vi "CoMP-S Logging To Text File.vi"(8 "error in (no error)":errorcluster, 9 "Oversizing":bool, 11 "Input text":string) -> (0 "error out":errorcluster)   [LabVIEW 2014]
panel:
  out "size (in bytes)":i64
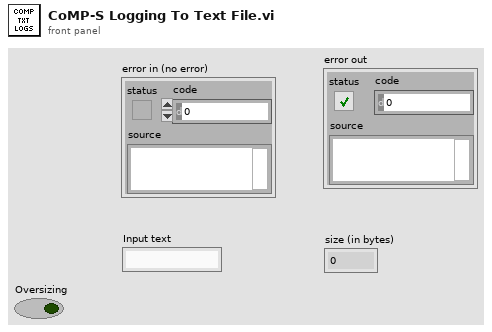
[diagram p1: front panel]
types:
  T1 = enum16{"open", "replace", "create", "open or create", "replace or create", "replace or create with confirmation"}
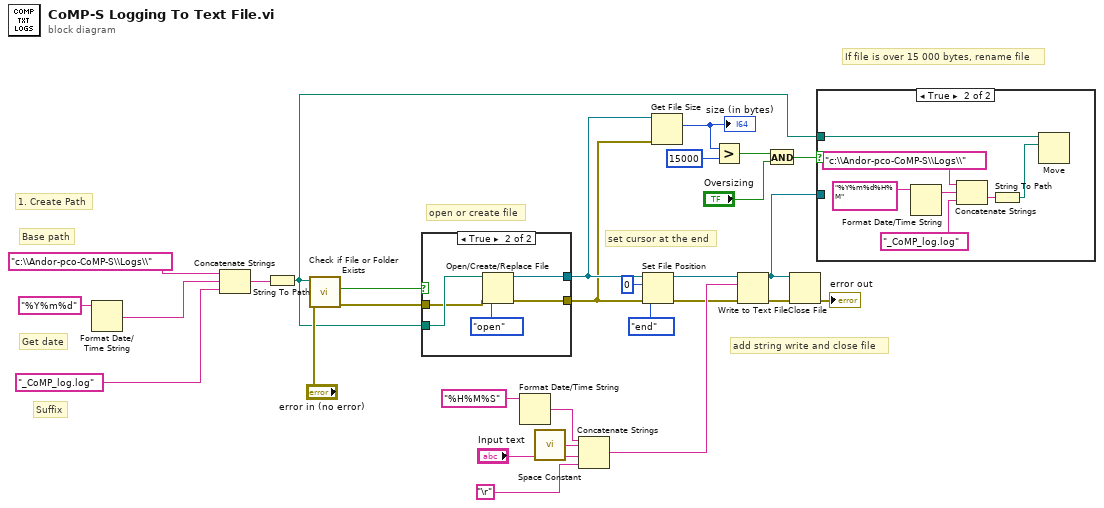
[diagram p0: block diagram]
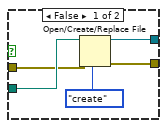
[diagram p3: hidden frame]
diagram:
  # "If file is over 15 000 bytes, rename file"
  # "set cursor at the end"
  # "open or create file"
  # "Suffix"
  # "1. Create Path"
  # "Get date"
  # "Base path"
  # "add string write and close file"
  n1 = Format Date/Time String(time format string (%c)="%Y%m%d") -> (date/time string=w4:string)  [unwired: 2 in]
  n2 = Concatenate Strings("c:\\Andor-pco-CoMP-S\\Logs\\" ("time format string (%c)"), w4, "_CoMP_log.log") -> (w26:string)
  n3 = String To Path(string=w26) -> (path=w9:path)
  n4 = call <vilib>:"Check if File or Folder Exists.vi"("error in (no error)"="error in (no error)", "path"=w9) -> ("error out"=w17:errorcluster, "file or folder exists?"=w25:bool)  [unwired: 7 in, 1 out]
  n5 = case shown="True" w25 {
    tunnel: w9 -> [w34 w38]
    tunnel: [w33 w37] -> w14
    tunnel: [w31 w36] -> w13
    tunnel: w17 -> [w30 w35]
    frame False {
      n6 = Open/Create/Replace File(file path (use dialog)=w34, error in=w30, operation (0:open)=T1."create") -> (refnum out=w33:refnum<file>, error out=w31:errorcluster)  [unwired: 3 in, 1 out]
    }
    frame True {
      n7 = Open/Create/Replace File(file path (use dialog)=w38, error in=w35, operation (0:open)=T1."open") -> (refnum out=w37:refnum<file>, error out=w36:errorcluster)  [unwired: 3 in, 1 out]
    }
  }
  n8 = Format Date/Time String(time format string (%c)="%H%M%S") -> (date/time string=w2:string)  [unwired: 2 in]
  n9 = call <vilib>:"Space Constant.vi"() -> ("String"=w1:string)
  n10 = Concatenate Strings(w2, w1, "Input text", "\r") -> (w19:string)
  n11 = Set File Position(offset (in bytes) (0)=i64 0, refnum=w14, from (0:start)=enum16{"start", "end", "current"}."end", error in=w13) -> (refnum out=w24:refnum<file>, error out=w18:errorcluster)
  n12 = Get File Size(file=w14, error in=w13) -> (size (in bytes)=w12:i64)  [unwired: 2 out]
  "size (in bytes)" <- w12
  n13 = Greater?(x=w12, y=i64 15000) -> (0:w8:bool)
  n14 = Write to Text File(file (use dialog)=w24, text=w19, error in=w18) -> (refnum out=w10:refnum<file>, error out=w29:errorcluster)  [unwired: 1 in, 1 out]
  n15 = And(x=w8, y="Oversizing") -> (x .and. y?=w7:bool)
  n16 = Close File(refnum=w10, error in=w29) -> (error out=→"error out":errorcluster)  [unwired: 1 out]
  n17 = case shown="True" w7 {
    tunnel: w10 -> [_ _]
    tunnel: w9 -> [_ w46]
    frame False {
    }
    frame True {
      n18 = Format Date/Time String(time format string (%c)="%Y%m%d%H%M") -> (date/time string=w40:string)  [unwired: 2 in]
      n19 = Concatenate Strings("c:\\Andor-pco-CoMP-S\\Logs\\", w40, "_CoMP_log.log" ("string")) -> (w44:string)
      n20 = String To Path(string=w44) -> (path=w43:path)
      n21 = Move(source path=w46, 10:w43) -> ()  [unwired: 3 in, 3 out]
    }
  }
